vi "digital_line_control_flow.vi"(8 "error in":errorcluster, 10 "ON/OFF":bool, 11 "lines 2":tag) -> (0 "error out":errorcluster)   [LabVIEW 2012]
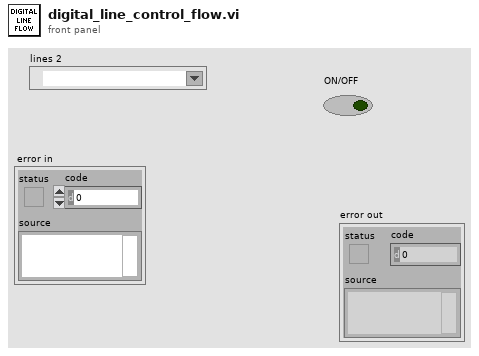
[diagram p1: front panel]
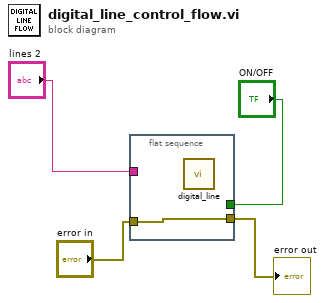
[diagram p0: block diagram]
diagram:
  n1 = flat-sequence {
    tunnel: [w8] -> w4
    tunnel: "error in" -> [w8]
    tunnel: "lines 2" -> [_]
    tunnel: "ON/OFF" -> [w6]
    frame #0 {
      n2 = call "digital_line.vi"() -> (2:w5, 3:w7)  [unwired: 5 in, 1 out]
    }
  }
  "error out" <- w4
